vi "_FPGA_Driver_LTC1667_3.vi"(7 "Enable":bool=TRUE, 8 "Clk":bool, 10 "Data_in":fxp<+,14,14>) -> ()   [LabVIEW 2018]
uses:
  <vilib>/rvi/eio/common/nirviEmuTemplateMethod_errors.vi
  <vilib>/eio/EIONode/EIONode.xnode
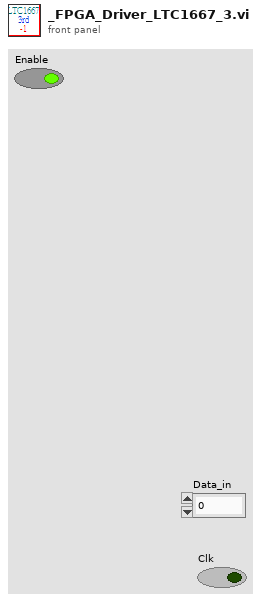
[diagram p1: front panel]
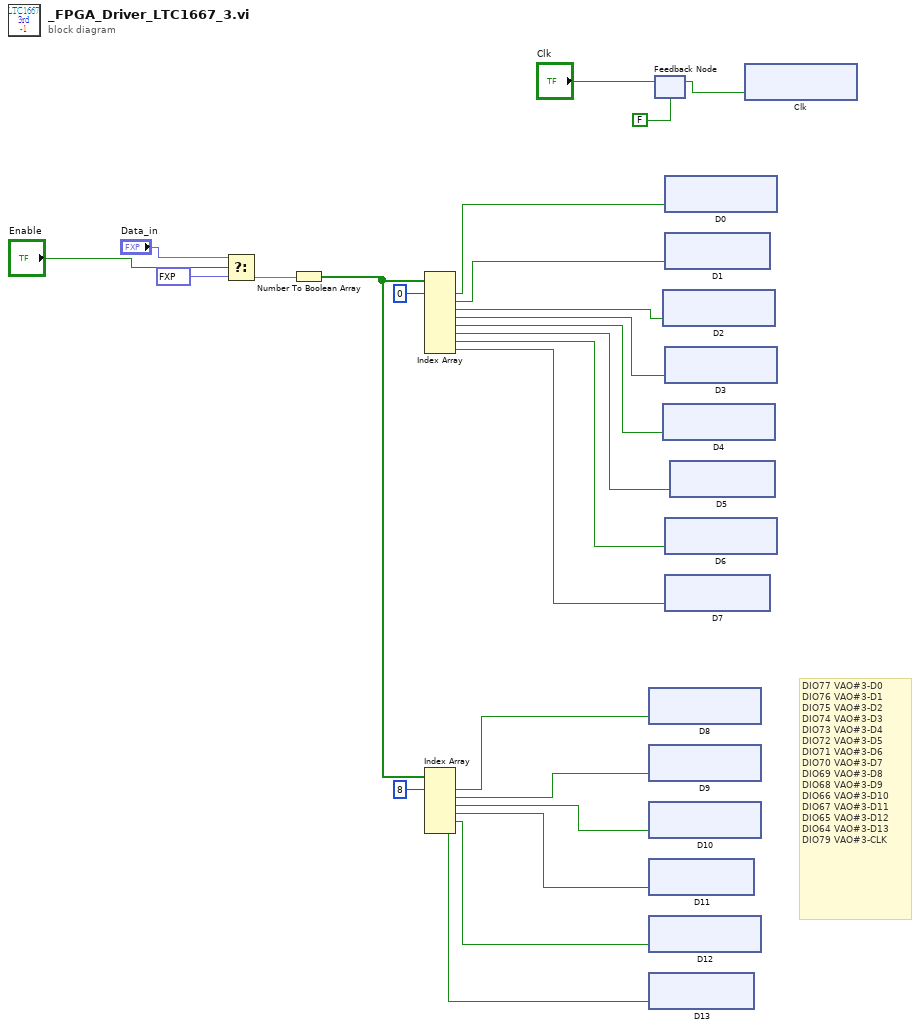
[diagram p0: block diagram]
diagram:
  # "DIO77\tVAO#3-D0\nDIO76\tVAO#3-D1\nDIO75\tVAO#3-D2\nDIO74\tVAO#3-D3\nDIO73\tVAO#3-D4\nDIO72\tVAO#3-D5\nDIO71\tVAO#3-D6\nDIO70\tVAO#3-D7\nDIO69\tVAO#3-D8\nDIO68\tVAO#3-D9\nDIO66\tVAO#3-D10\nDIO67\tVAO#3-D11\nDIO65\tVAO#3-D12\nDIO64\tVAO#3-D13\nDIO79\tVAO#3-CLK"
  n1 = Select(t="Data_in", s="Enable", f=fxp<+,14,14> 8192.0) -> (s? t:f=w19:fxp<+,14,14>)
  n2 = Number To Boolean Array(number=w19) -> (Boolean array=w22:bool[])
  n3 = Index Array(array=w22, index #1=0 ("index")) -> (element #1=w15:bool, element #2=w14:bool, element #3=w13:bool, element #4=w12:bool, element #5=w11:bool, element #6=w10:bool, element #7=w9:bool, element #8=w8:bool)  [unwired: 7 in]
  n4 = Index Array(array=w22, index #1=8 ("index")) -> (element #1=w6:bool, element #2=w5:bool, element #3=w4:bool, element #4=w3:bool, element #5=w2:bool, element #6=w1:bool)  [unwired: 5 in]
  n5 = xnode "D8"("RMC/DIO67"=w6) -> ()  [unwired: 1 in, 1 out]
  n6 = xnode "D9"("RMC/DIO34"=w5) -> ()  [unwired: 1 in, 1 out]
  n7 = xnode "D10"("RMC/DIO66"=w4) -> ()  [unwired: 1 in, 1 out]
  n8 = xnode "D11"("RMC/DIO2"=w3) -> ()  [unwired: 1 in, 1 out]
  n9 = xnode "D12"("RMC/DIO33"=w2) -> ()  [unwired: 1 in, 1 out]
  n10 = xnode "D13"("RMC/DIO1"=w1) -> ()  [unwired: 1 in, 1 out]
  n11 = feedback-in #1("Clk") -> ()
  n12 = feedback #1(FALSE ("Clk")) -> (w7:bool)
  n13 = xnode "D2"("RMC/DIO69"=w13) -> ()  [unwired: 1 in, 1 out]
  n14 = xnode "D4"("RMC/DIO68"=w11) -> ()  [unwired: 1 in, 1 out]
  n15 = xnode "D0"("RMC/DIO77"=w15) -> ()  [unwired: 1 in, 1 out]
  n16 = xnode "D1"("RMC/DIO5"=w14) -> ()  [unwired: 1 in, 1 out]
  n17 = xnode "D3"("RMC/DIO36"=w12) -> ()  [unwired: 1 in, 1 out]
  n18 = xnode "D6"("RMC/DIO35"=w9) -> ()  [unwired: 1 in, 1 out]
  n19 = xnode "D7"("RMC/DIO3"=w8) -> ()  [unwired: 1 in, 1 out]
  n20 = xnode "D5"("RMC/DIO4"=w10) -> ()  [unwired: 1 in, 1 out]
  n21 = xnode "Clk"("RMC/DIO65"=w7) -> ()  [unwired: 1 in, 1 out]
